vi "ni_move_backlash.vi"(6 "Axis enable":bool[](array[boolean])=[TRUE, TRUE, TRUE, TRUE], 8 "error in":errorcluster, 9 "Axis positions":dbl[](array[numeric]), 10 "Absolute":bool=TRUE) -> (0 "error out":errorcluster)   [LabVIEW 2011]
panel:
  out "Pull-in errors":i32[][](graph)
  out "Pull in iterations":i32
  in  "Pull in gain":dbl=1.0
  in  "Clear histogram":bool
  out "Final axis errors":i32[](array[numeric])
  in  "Histogram N":i32=10
  out "Error histogram":cluster{"X":i32[], "Y":i32[]}[](graph)
  in  "Pull in offset":i32=15
  in  "Backlash offset":i32=40
  # "Diagnostics"
  # "The controller axis numbers (starting from 1)"
  # "Like ni_move.vi, but always approaches the position in the + direction.  This minimizes the contribution of backlash to nonrepeatability.  For this to work, pull-in moves must be set to 0 for the axes so that the motion controller won't try to back up."
  # "Parameters:"
  # "Amount we offset position by when approaching from the reverse direction.  Some value greater than the backlash (in steps.)"
  # "Amount we stop short in direction of travel.  Some value (in steps) more than the typical open-loop error, but well less than a full step.  This way our pull-in move is always in the right direction."
  # "Fraction of remaining distance we pull in on each move.   It seeems\nwe always undershoot, so gain = 1."
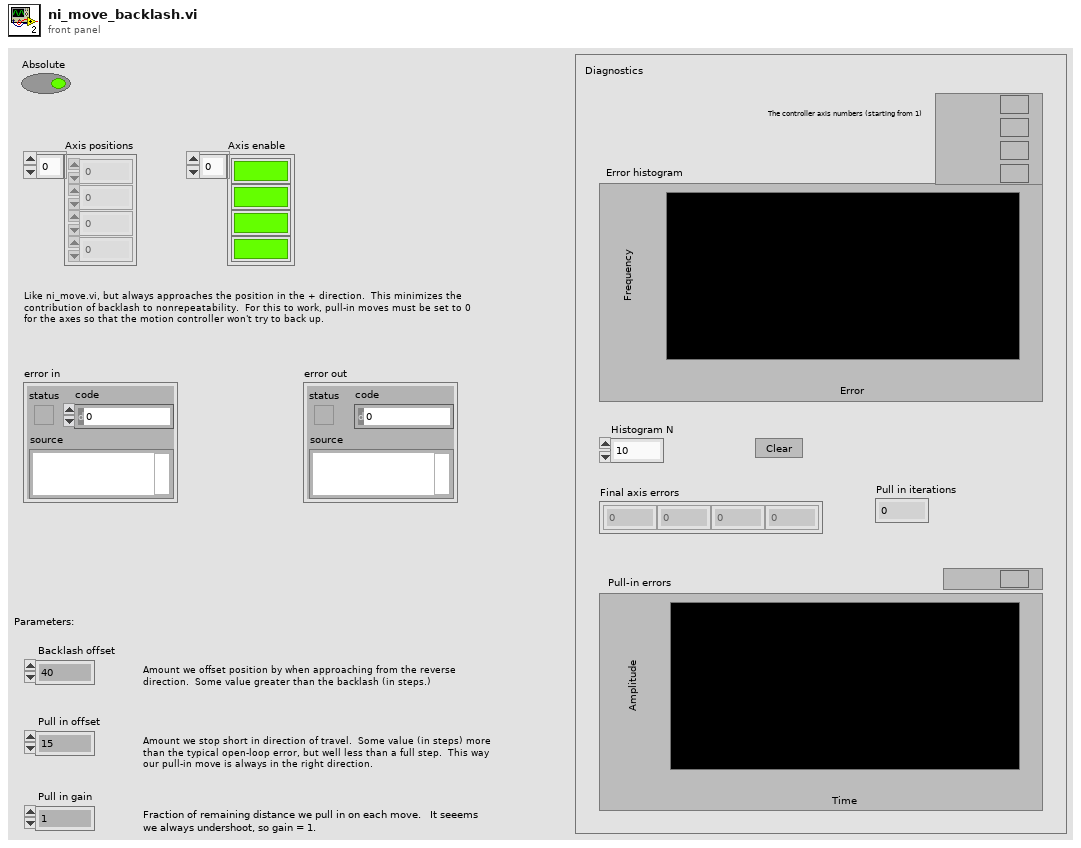
[diagram p1: front panel]
types:
  T1 = typedef "Board Id" = u8
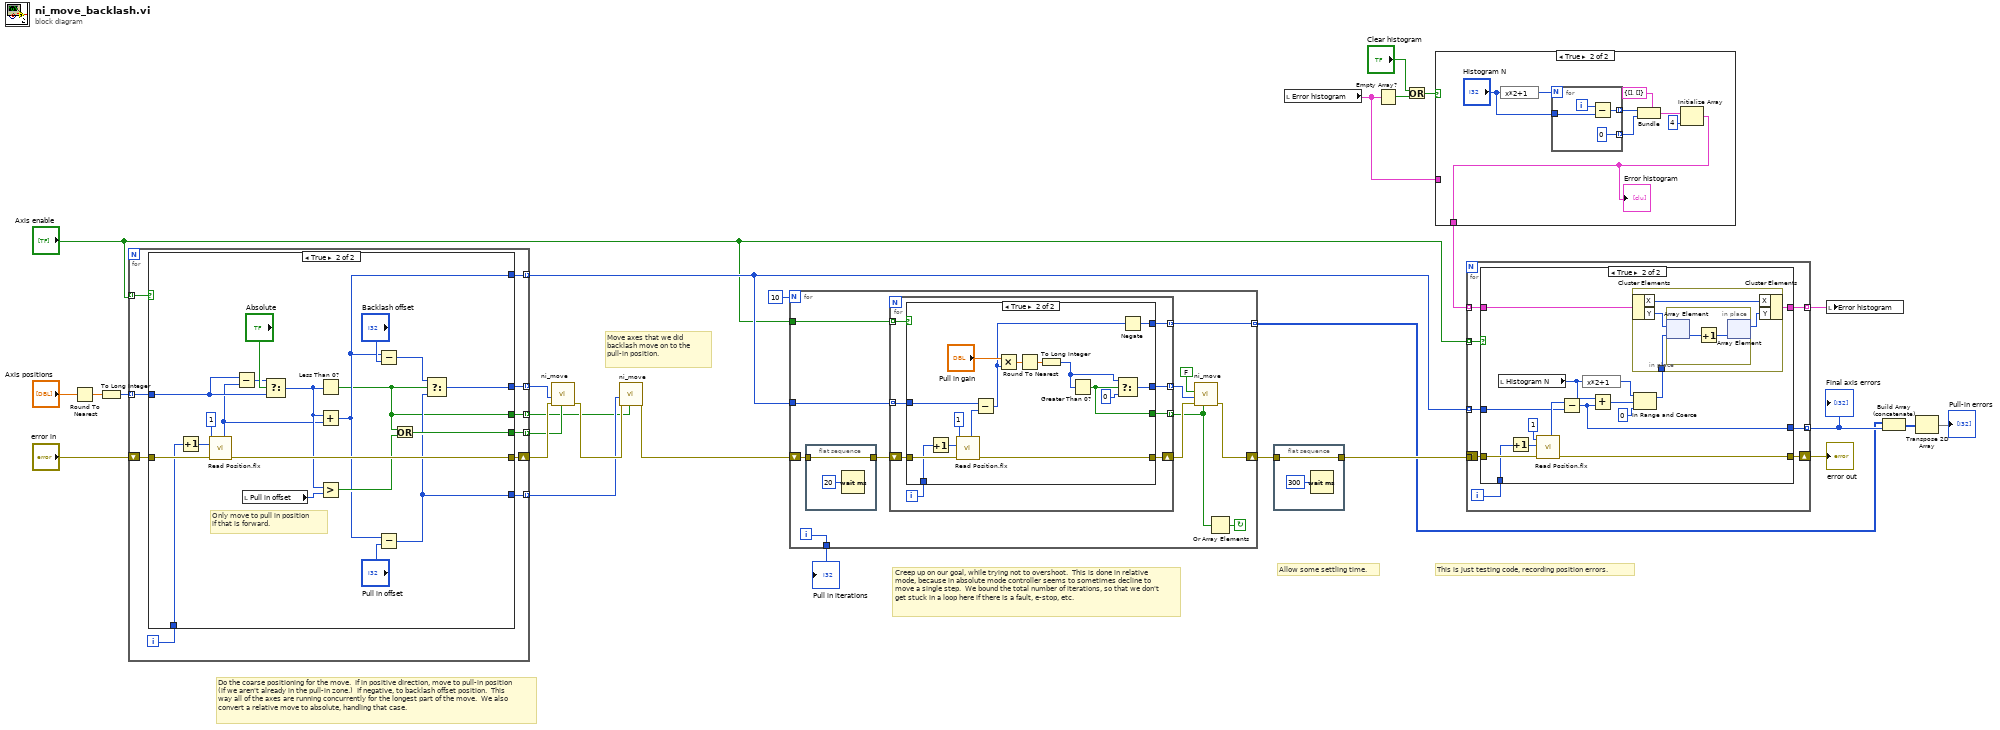
[diagram p0: block diagram]
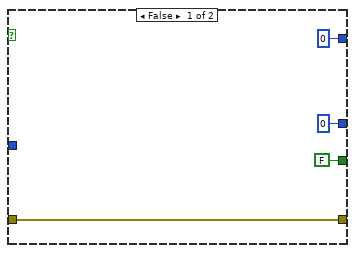
[diagram p2: hidden frame]
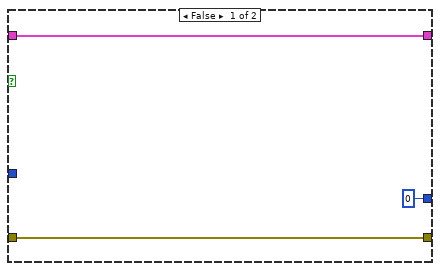
[diagram p4: hidden frame]
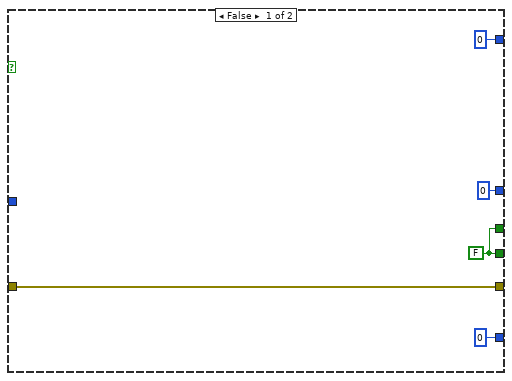
[diagram p5: hidden frame]
diagram:
  # "Allow some settling time."
  # "Creep up on our goal, while trying not to overshoot.  This is done in relative mode, because in absolute mode controller seems to sometimes decline to move a single step.  We bound the total number of iterations, so that we don't get stuck in a loop here if there is a fault, e-stop, etc."
  # "This is just testing code, recording position errors."
  # "Move axes that we did backlash move on to the pull-in position."
  # "Do the coarse positioning for the move.  If in positive direction, move to pull-in position (if we aren't already in the pull-in zone.)  If negative, to backlash offset position.  This way all of the axes are running concurrently for the longest part of the move.  We also convert a relative move to absolute, handling that case."
  n1 = Round To Nearest(number="Axis positions") -> (nearest integer value=w27:dbl[])
  n2 = To Long Integer(number=w27) -> (32bit integer=w25:i32[])
  n3 = for {
    tunnel: "Axis enable" -> [w37] mode=indexing
    tunnel: w25 -> [w36] mode=indexing
    shift-right: [w35] -> w23
    shift-left: "error in" -> [w38]
    tunnel: [w33] -> w3 mode=indexing
    tunnel: [w32] -> w21 mode=indexing
    tunnel: [w31] -> w24 mode=indexing
    tunnel: [w30] -> w2 mode=indexing
    tunnel: [w29] -> w1 mode=indexing
    i -> [w34]
    n4 = case shown="True" w37 {
      tunnel: w38 -> [w43 w62]
      tunnel: w34 -> [_ w57]
      tunnel: w36 -> [_ w59]
      tunnel: [w43 w58] -> w35
      tunnel: [w40 w51] -> w33
      tunnel: [0 w48] -> w32
      tunnel: [0 w46] -> w31
      tunnel: [0 w45] -> w30
      tunnel: [w40 w44] -> w29
      frame False {
        w40 = FALSE
      }
      frame True {
        # "Only move to pull in position\nif that is forward."
        n5 = Increment(x=w57) -> (x+1=w56:i32)
        n6 = call <vilib>:"Read Position.flx"("error in (no error)"=w62, "Axis"=w56, "Board ID"=T1 1) -> ("error out"=w58:errorcluster, "Position"=w49:i32)  [unwired: 3 in, 2 out]
        n7 = Subtract(x=w59, y=w49) -> (x-y=w60:i32)
        n8 = local read "Pull in offset"() -> (w54:i32)
        n9 = Select(t=w60, s="Absolute", f=w59) -> (s? t:f=w52:i32)
        n10 = Less Than 0?(x=w52) -> (x < 0?=w44:bool)
        n11 = Add(x=w52, y=w49) -> (x+y=w48:i32)
        n12 = Greater?(x=w52, y=w54) -> (0:w53:bool)
        n13 = Subtract(x=w48, y="Backlash offset") -> (x-y=w47:i32)
        n14 = Subtract(x=w48, y="Pull in offset") -> (x-y=w45:i32)
        n15 = Or(x=w44, y=w53) -> (x .or. y?=w51:bool)
        n16 = Select(t=w47, s=w44, f=w45) -> (s? t:f=w46:i32)
      }
    }
  }
  n17 = call "ni_move.vi"("Axis enable"=w3, "error in"=w23, "Axis positions"=w24) -> ("error out"=w22:errorcluster)  [unwired: 8 in]
  n18 = call "ni_move.vi"("Axis enable"=w1, "error in"=w22, "Axis positions"=w2) -> ("error out"=w9:errorcluster)  [unwired: 8 in]
  n19 = for {
    N: 10 -> [_]
    tunnel: "Axis enable" -> [w73]
    tunnel: w21 -> [w72]
    tunnel: [w69] -> w12
    tunnel: [w64] -> w5 mode=indexing
    shift-right: [w71] -> w17
    shift-left: w9 -> [w66]
    i -> [w69]
    stop <- w68 continue-if-true
    n20 = flat-sequence {
      tunnel: w66 -> [w76]
      tunnel: [w76] -> w65
      frame #0 {
        n21 = Wait (ms)(milliseconds to wait=u32 20) -> ()  [unwired: 1 out]
      }
    }
    n22 = for {
      tunnel: w73 -> [w84] mode=indexing
      tunnel: w72 -> [w83] mode=indexing
      shift-right: [w82] -> w75
      shift-left: w65 -> [w85]
      tunnel: [w80] -> w70 mode=indexing
      tunnel: [w79] -> w74 mode=indexing
      tunnel: [w78] -> w64 mode=indexing
      i -> [w81]
      n23 = case shown="True" w84 {
        tunnel: w85 -> [w89 w103]
        tunnel: w81 -> [_ w99]
        tunnel: w83 -> [_ w97]
        tunnel: [w89 w102] -> w82
        tunnel: [FALSE w105] -> w80
        tunnel: [0 w101] -> w79
        tunnel: [0 w90] -> w78
        frame False {
        }
        frame True {
          n24 = Increment(x=w99) -> (x+1=w98:i32)
          n25 = call <vilib>:"Read Position.flx"("error in (no error)"=w103, "Axis"=w98, "Board ID"=T1 1) -> ("error out"=w102:errorcluster, "Position"=w95:i32)  [unwired: 3 in, 2 out]
          n26 = Subtract(x=w97, y=w95) -> (x-y=w91:i32)
          n27 = Multiply(x="Pull in gain", y=w91) -> (x*y=w94:dbl)
          n28 = Round To Nearest(number=w94) -> (nearest integer value=w93:dbl)
          n29 = To Long Integer(number=w93) -> (32bit integer=w92:i32)
          n30 = Greater Than 0?(x=w92) -> (x > 0?=w105:bool)
          n31 = Select(t=w92, s=w105, f=0) -> (s? t:f=w101:i32)
          n32 = Negate(x=w91) -> (-x=w90:i32)
        }
      }
    }
    n33 = call "ni_move.vi"("Axis enable"=w70, "error in"=w75, "Axis positions"=w74, "Absolute"=FALSE) -> ("error out"=w71:errorcluster)  [unwired: 7 in]
    n34 = Or Array Elements(Boolean array=w70) -> (logical OR=w68:bool)
  }
  "Pull in iterations" <- w12
  n35 = flat-sequence {
    tunnel: w17 -> [w106]
    tunnel: [w106] -> w16
    frame #0 {
      n36 = Wait (ms)(milliseconds to wait=u32 300) -> ()  [unwired: 1 out]
    }
  }
  n37 = local read "Error histogram"() -> (w20:cluster{"X":i32[], "Y":i32[]}[])
  n38 = Empty Array?(array=w20) -> (empty?=w14:bool)
  n39 = Or(x="Clear histogram", y=w14) -> (x .or. y?=w13:bool)
  n40 = case shown="True" w13 {
    tunnel: w20 -> [w108 _]
    tunnel: [w108 w109] -> w19
    frame False {
      # "Histogram initialized"
    }
    frame True {
      n41 = expression code="x*2+1"("Histogram N") -> (w116:i32)
      n42 = for {
        N: w116 -> [_]
        tunnel: "Histogram N" -> [w119]
        tunnel: [w118] -> w114 mode=indexing
        tunnel: [0 ("Histogram N")] -> w113 mode=indexing
        i -> [w120]
        n43 = Subtract(x=w120, y=w119) -> (x-y=w118:i32)
      }
      n44 = Bundle(cluster=cluster{"X":i32[], "Y":i32[]} {"X"=[], "Y"=[]}, "X"=w114, "Y"=w113) -> (w112:cluster{"X":i32[], "Y":i32[]})
      n45 = Initialize Array(w112, 4 ("dimension size")) -> (w109:cluster{"X":i32[], "Y":i32[]}[])
      "Error histogram" <- w109
    }
  }
  n46 = for {
    tunnel: "Axis enable" -> [w127] mode=indexing
    tunnel: w21 -> [w126] mode=indexing
    shift-right: [w125] -> w18
    shift-left: _ -> [w128]
    tunnel: w19 -> [w123] mode=indexing
    tunnel: [w122] -> w10 mode=indexing
    tunnel: w16 -> [_]
    tunnel: [w121] -> w8 mode=indexing
    i -> [w124]
    n47 = case shown="True" w127 {
      tunnel: w128 -> [w131 w145]
      tunnel: w124 -> [_ w137]
      tunnel: w126 -> [_ w135]
      tunnel: [w131 w144] -> w125
      tunnel: w123 -> [w130 w141]
      tunnel: [w130 w139] -> w122
      tunnel: [0 w134] -> w121
      frame False {
      }
      frame True {
        n48 = local read "Histogram N"() -> (w133:i32)
        n49 = Increment(x=w137) -> (x+1=w138:i32)
        n50 = call <vilib>:"Read Position.flx"("error in (no error)"=w145, "Axis"=w138, "Board ID"=T1 1) -> ("error out"=w144:errorcluster, "Position"=w136:i32)  [unwired: 3 in, 2 out]
        n51 = Subtract(x=w136, y=w135) -> (x-y=w134:i32)
        n52 = expression code="x*2+1"(w133) -> (w132:i32)
        n53 = Add(x=w133, y=w134) -> (x+y=w143:i32)
        n54 = In Range and Coerce(upper limit=w132, x=w143, lower limit=0) -> (coerced(x)=w140:i32)  [unwired: 1 out]
        n55 = in-place {
          in-place-border: w140 -> [w148]
          n56 = in-place-cluster #1(w141) -> ("X"=w150:i32[], "Y"=w149:i32[])
          n57 = in-place {
            n58 = in-place-array #2(w149, w148) -> (w152:i32)
            n59 = Increment(x=w152) -> (x+1=w151:i32)
            n60 = in-place-array #2(w151) -> (w147:i32[])  [unwired: 1 out]
          }
          n61 = in-place-cluster #1("X"=w150, "Y"=w147) -> (w139:cluster{"X":i32[], "Y":i32[]})
        }
      }
    }
  }
  "error out" <- w18
  "Final axis errors" <- w8
  n62 = local write "Error histogram"(w10) -> ()
  n63 = Build Array (concatenate)(w5, w8) -> (w7:i32[][])
  n64 = Transpose 2D Array(2D array=w7) -> (transposed array=→"Pull-in errors":i32[][])
